vi "Integer to Diode Current.vi"(11 "Current Int":i16) -> (3 "Current (mA)":dbl)   [LabVIEW 2016, in "Laser Diode Controller.lvlib" / "KLD101.lvclass"]
uses:
  KLD101.lvclass
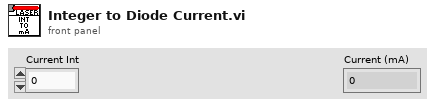
[diagram p1: front panel]
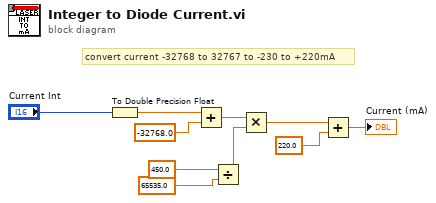
[diagram p0: block diagram]
diagram:
  # "convert current -32768 to 32767 to -230 to +220mA"
  n1 = To Double Precision Float(number="Current Int") -> (double precision float=w1:dbl)
  n2 = Add(x=w1, y=-32768.0) -> (x+y=w6:dbl)
  n3 = Divide(x=450.0 ("y"), y=65535.0) -> (x/y=w4:dbl)
  n4 = Multiply(x=w6, y=w4) -> (x*y=w5:dbl)
  n5 = Add(x=w5, y=220.0) -> (x+y=→"Current (mA)":dbl)
